vi "fit labview-Rev5.vi"(0 "modelname":string, 1 "B":dbl[](array[numeric])=array[4097 elements], 2 "y":dbl[](array[numeric])=array[4097 elements], 3 "npts":i32, 4 "modFreq":dbl, 5 "modAmp":dbl, 6 "pars":dbl[](array[numeric])=array[4097 elements], 7 "error in (no error)":errorcluster, 8 "parsError":dbl[](array[numeric])=array[4097 elements], 9 "vpp":dbl[](array[numeric])=array[4097 elements], 10 "ncomps":i32, 11 "fit":dbl[](array[numeric])=array[4097 elements]) -> (16 "ncomps out":i32, 17 "fit out":dbl[](array[numeric]), 18 "parsError out":dbl[](array[numeric]), 19 "vpp out":dbl[](array[numeric]), 26 "pars out":dbl[](array[numeric]), 27 "error out":errorcluster)   [LabVIEW 2016, in "libFitSpectraLabview_Rev5.lvlib"]
doc: "void FIT_LABVIEW_API fit_labview(const char *modelname,\n const double *B, const double *y,\n const int *npts, const double *modFreq, const double *modAmp,\n double *pars, double *parsError, double *vpp, int *ncomps, double *fit);"
uses:
  libFitSpectraLabview_Rev5.lvlib
  Documents/Software/Labview Fitting/LabviewCompiled/Rev5/libFitSpectraLabview_Rev5.dll
panel:
  # "test"
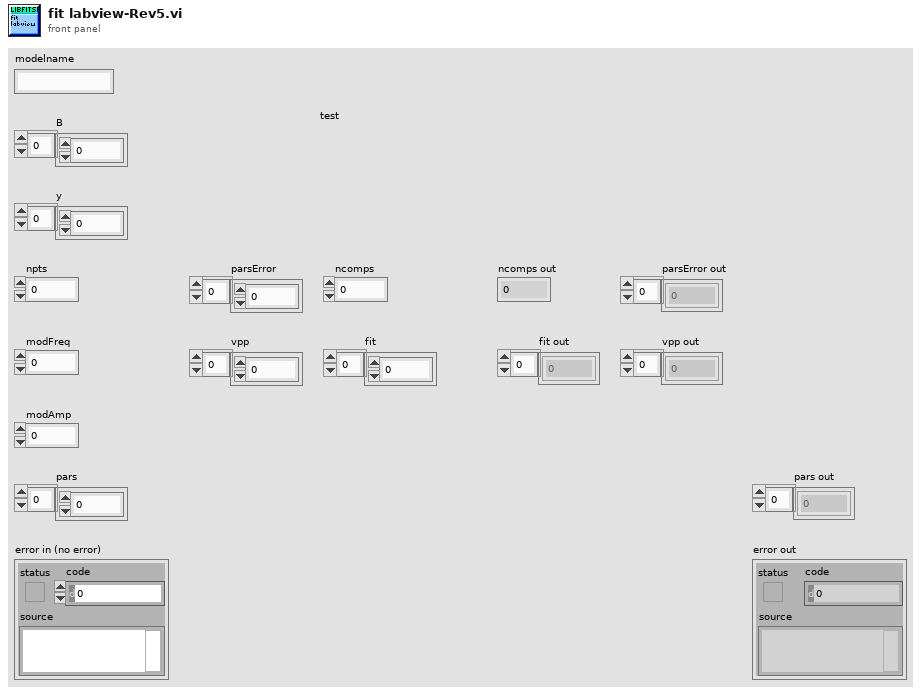
[diagram p1: front panel]
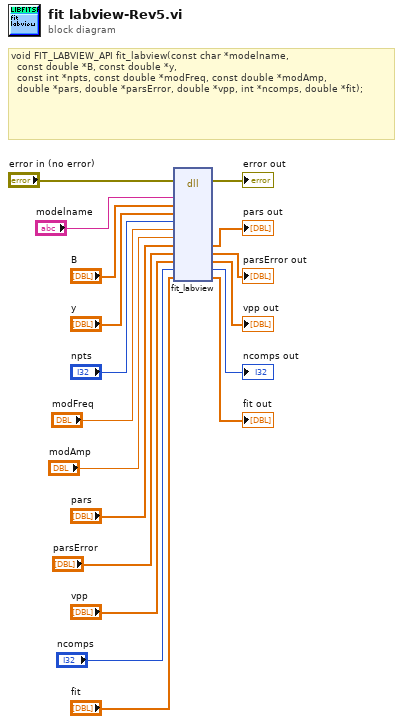
[diagram p0: block diagram]
diagram:
  # "void FIT_LABVIEW_API fit_labview(const char *modelname,\n\t\tconst double *B, const double *y,\n\t\tconst int *npts, const double *modFreq, const double *modAmp,\n\t\tdouble *pars, double *parsError, double *vpp, int *ncomps, double *fit);"
  n1 = dll-call lib="C:/Users/Wilson Schreiber/Documents/Software/Labview Fitting/LabviewCompiled/Rev5/libFitSpectraLabview_Rev5.*" fn="fit_labview"(error in="error in (no error)", "modelname"="modelname", "B"="B", "y"="y", "npts"="npts", "modFreq"="modFreq", "modAmp"="modAmp", "pars"="pars", "parsError"="parsError", "vpp"="vpp", "ncomps"="ncomps", "fit"="fit") -> (error out=→"error out":errorcluster, "pars"=→"pars out":dbl[], "parsError"=→"parsError out":dbl[], "vpp"=→"vpp out":dbl[], "ncomps"=→"ncomps out":i32, "fit"=→"fit out":dbl[])  [unwired: 9 in, 1 out]
